vi "SampleGetIDMultiple_8742.vi"() -> ()   [LabVIEW 2009]
panel:
  out "Identification List":string[](array[string])
  out "DeviceKey List Out":string[](array[string])
  out "error out":errorcluster
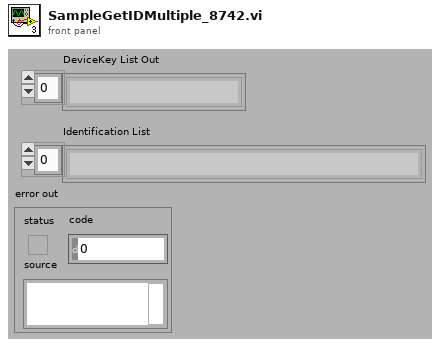
[diagram p1: front panel]
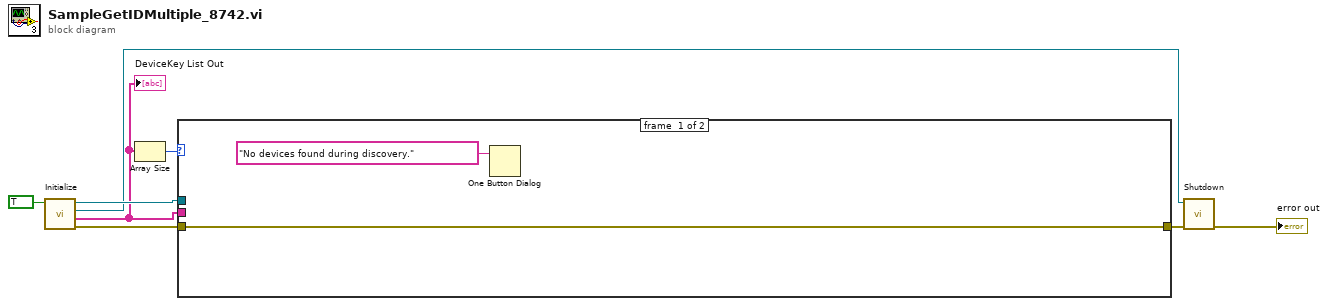
[diagram p0: block diagram]
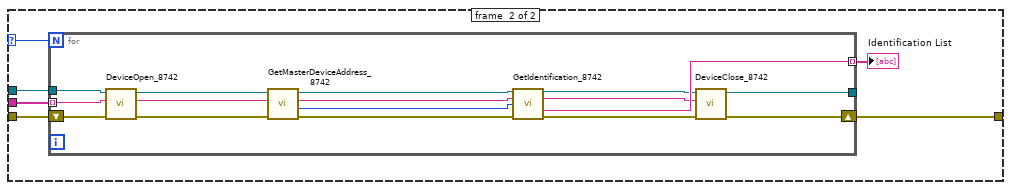
[diagram p2: hidden frame]
diagram:
  n1 = call "Initialize.vi"("logging"=TRUE) -> ("error out"=w4:errorcluster, "DeviceKey List"=w2:string[], "DeviceIOLib Out"=w1:refnum<k24>, "CmdLib Out"=w5:refnum<k24>)  [unwired: 3 in]
  "DeviceKey List Out" <- w2
  n2 = Array Size(array=w2) -> (size(s)=w6:i32)
  n3 = case shown="1, Default" w6 {
    selector: w6 -> [_ w16]
    tunnel: w2 -> [_ w15]
    tunnel: w5 -> [_ w14]
    tunnel: w4 -> [w10 w13]
    tunnel: [w10 w12] -> w3
    frame #0 {
      n4 = One Button Dialog(message="No devices found during discovery.") -> ()  [unwired: 1 in, 1 out]
    }
    frame #1 {
      n5 = for {
        N: w16 -> [_]
        tunnel: w15 -> [w28] mode=indexing
        tunnel: [w32] -> w11 mode=indexing
        tunnel: w14 -> [w31]
        tunnel: [w30] -> _
        shift-right: [w26] -> w12
        shift-left: w13 -> [w27]
        n6 = call "DeviceOpen_8742.vi"("error in (no error)"=w27, "DeviceKey In"=w28, "CmdLib In"=w31) -> ("error out"=w21:errorcluster, "DeviceKey Out"=w22:string, "CmdLib Out"=w23:refnum<k24>)  [unwired: 2 in]
        n7 = call "GetMasterDeviceAddress_8742.vi"("error in (no error)"=w21, "DeviceKey In"=w22, "CmdLib In"=w23) -> ("error out"=w17:errorcluster, "Device Address"=w20:i32, "DeviceKey Out"=w19:string, "CmdLib Out"=w18:refnum<k24>)  [unwired: 1 in]
        n8 = call "GetIdentification_8742.vi"("CmdLib In"=w18, "DeviceKey In"=w19, "Device Address In"=w20, "error in (no error)"=w17) -> ("CmdLib Out"=w29:refnum<k24>, "DeviceKey Out"=w24:string, "Identification"=w32:string, "error out"=w25:errorcluster)  [unwired: 7 in, 1 out]
        n9 = call "DeviceClose_8742.vi"("error in (no error)"=w25, "DeviceKey In"=w24, "CmdLib In"=w29) -> ("error out"=w26:errorcluster, "CmdLib Out"=w30:refnum<k24>)  [unwired: 2 in, 1 out]
      }
      "Identification List" <- w11
    }
  }
  n10 = call "Shutdown.vi"("error in (no error)"=w3, "DeviceIOLib In"=w1) -> ("error out"=→"error out":errorcluster)  [unwired: 5 in]
